vi "Init.vi"(10 "Setup":T1) -> (3 "Base Setup out":refnum<class "Base Setup.lvclass">)   [LabVIEW 2025, in "jettl.lvlib" / "Setup.lvlib" / "Base Setup.lvclass"]
uses:
  Base Setup.lvclass
  Setup.ctl
  Attributes/Attributes/Attributes.lvclass
  Transport/Transport/Transport.lvclass
  Msg Set.ctl
  Msg/Msg.lvclass
  Actor/Actor.lvclass
  Base Setup.lvclass/Base Setup.ctl
  jettl.lvlib
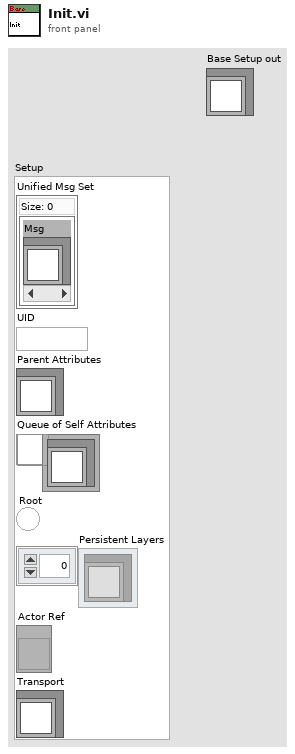
[diagram p1: front panel]
types:
  T1 = typedef "jettl.lvlib/Setup.ctl" = cluster{"Unified Msg Set":T2, "UID":string, "Parent Attributes":refnum<class "Attributes.lvclass">, "Queue of Self Attributes":refnum<queue>, "Root":bool, "Persistent Layers":refnum<class "Actor.lvclass">[], "Actor Ref":refnum<vi>, "Transport":refnum<class "Transport.lvclass">}
  T2 = typedef "jettl.lvlib/Msg Set.ctl" = set{refnum<class "Msg.lvclass">}
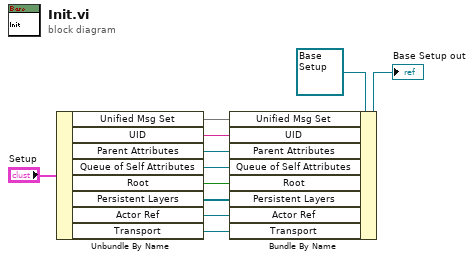
[diagram p0: block diagram]
diagram:
  n1 = Unbundle By Name("Setup") -> ("Unified Msg Set"=w8:T2, "UID"=w7:string, "Parent Attributes"=w6:refnum<class "Attributes.lvclass">, "Queue of Self Attributes"=w5:refnum<queue>, "Root"=w4:bool, "Persistent Layers"=w3:refnum<class "Actor.lvclass">[], "Actor Ref"=w2:refnum<vi>, "Transport"=w1:refnum<class "Transport.lvclass">)
  n2 = Bundle By Name(cluster=refnum<class "Base Setup.lvclass"> refnum ("Base Setup out"), "Unified Msg Set"=w8, "UID"=w7, "Parent Attributes"=w6, "Queue of Self Attributes"=w5, "Root"=w4, "Persistent Layers"=w3, "Actor Ref"=w2, "Transport"=w1) -> (→"Base Setup out":refnum<class "Base Setup.lvclass">)
